vi "Actor Core.vi"(8 "error in":errorcluster, 11 "ServiceManager in":refnum<class "ServiceManager.lvclass">) -> (0 "error out":errorcluster, 3 "Actor out":refnum<class "Actor.lvclass">)   [LabVIEW 2020, in "ServiceManager.lvlib" / "ServiceManager.lvclass"]
doc: "(<B>Filename</B>: Actor Framework.lvlib:Actor.lvclass:Actor Core.vi)\n\nReceives messages to the actor, reacts to them, and initiates any error handling that may shut the actor down.\n\nDescendant classes may override this VI to append parallel tasks for the actor to complete while it handles messages. Overrides use the Call Parent Class Method node."
uses:
  ServiceManager.lvclass
  C:/Program Files (x86)/National Instruments/LabVIEW 2020/vi.lib/ActorFramework/Actor/Actor.lvclass
  <vilib>/ActorFramework/Actor/Actor.lvclass
  ServiceManager.lvclass/ServiceManager.ctl
  ServiceManager-Comms/ServiceManager-Comms.lvclass
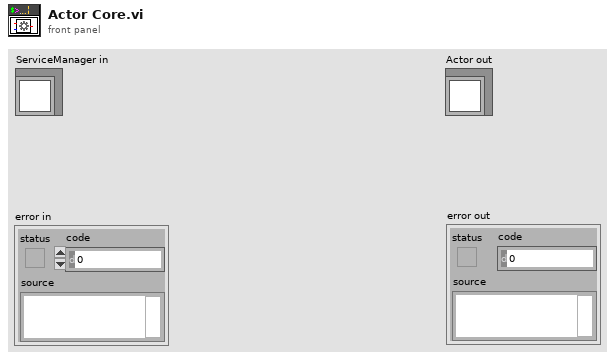
[diagram p1: front panel]
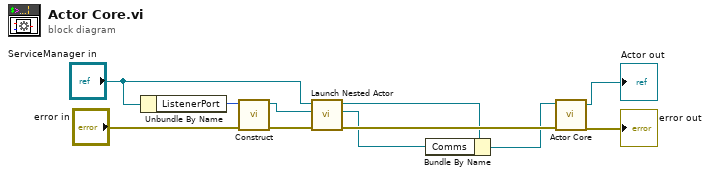
[diagram p0: block diagram]
diagram:
  n1 = Unbundle By Name("ServiceManager in") -> ("ListenerPort"=w7:u16)
  n2 = call "Construct.vi"("error in (no error)"="error in", "ListenerPort"=w7) -> ("error out"=w5:errorcluster, "ServiceManager-Comms out"=w4:refnum<class "ServiceManager-Comms.lvclass">)  [unwired: 8 in]
  n3 = call <vilib>:"Launch Nested Actor.vi"("error in (no error)"=w5, "Nested Actor"=w4, "Caller Actor in"="ServiceManager in") -> ("error out"=w9:errorcluster, "Nested Actor's Enqueuer"=w1:refnum<class "Message Enqueuer.lvclass">, "Caller Actor out"=w2:refnum<class "ServiceManager.lvclass">)  [unwired: 6 in]
  n4 = Bundle By Name(cluster=w2, "Comms"=w1) -> (w3:refnum<class "ServiceManager.lvclass">)
  n5 = call-parent "Actor Core.vi"("error in"=w9, "Actor in"=w3) -> ("error out"=→"error out":errorcluster, "Actor out"=→"Actor out":refnum<class "Actor.lvclass">)  [unwired: 8 in]
